vi "AppendStateToError.vi"(5 "error in":errorcluster, 6 "State":string) -> (19 "error out":errorcluster)   [LabVIEW 2020, in "G#IDE.lvlib" / "SupportLib.lvlib"]
uses:
  SupportLib.lvlib
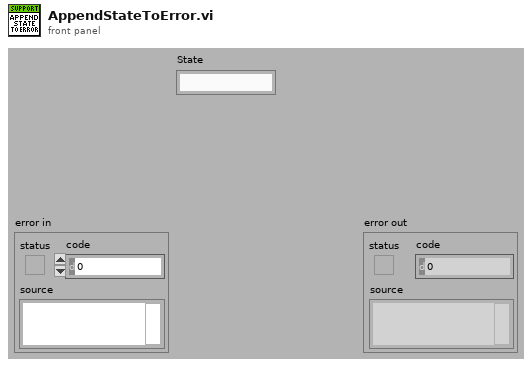
[diagram p1: front panel]
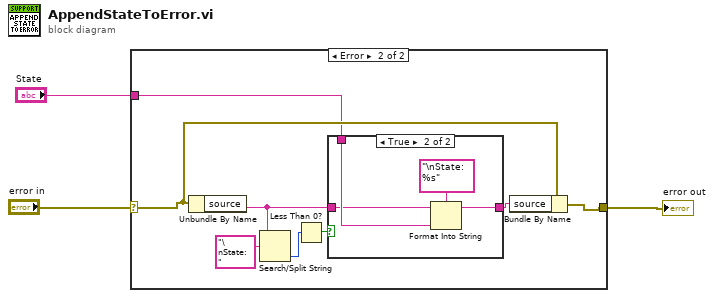
[diagram p0: block diagram]
diagram:
  n1 = case shown="Error" "error in" {
    selector: "error in" -> [w4 w12]
    tunnel: [w4 w11] -> w2
    tunnel: "State" -> [_ w10]
    frame No Error {
    }
    frame Error {
      n2 = Unbundle By Name(w12) -> ("source"=w6:string)
      n3 = Search/Split String(string=w6, search string/char (-)="\nState: " ("format string")) -> (offset of match=w7:i32)  [unwired: 1 in, 2 out]
      n4 = Less Than 0?(x=w7) -> (x < 0?=w5:bool)
      n5 = case shown="True" w5 {
        tunnel: w10 -> [_ w17]
        tunnel: [w13 w16] -> w9
        tunnel: w6 -> [w13 w14]
        frame False {
        }
        frame True {
          n6 = Format Into String(format string="\nState: %s", initial string=w14, w17) -> (resulting string=w16:string)  [unwired: 1 in, 1 out]
        }
      }
      n7 = Bundle By Name(cluster=w12, "source"=w9) -> (w11:errorcluster)
    }
  }
  "error out" <- w2
